vi "Filter_Lowpass - 2D.vi"(1 "Filter":bool caption="Scan", 2 "Input 2D":dbl[][](array[numeric]), 3 "low cutoff freq: fl":dbl=40.0 format="%0.2f") -> (7 "Output":dbl[][](array[numeric]))   [LabVIEW 2018]
uses:
  <vilib>/Analysis/3filter.llb/Filter Passband Type.ctl
  <vilib>/Analysis/4window.llb/windowTd.ctl
  <vilib>/Analysis/3filter.llb/FIR Windowed Filter (DBL).vi
  <vilib>/Analysis/NI_AALBase.lvlib
  <vilib>/Analysis/NI_AALPro.lvlib
  <vilib>/Platform/NI_3dgraph.lvlib
panel:
  in  "3D Surface 2":refnum<k7>(container)
  in  "3D Surface":refnum<k7>(container)
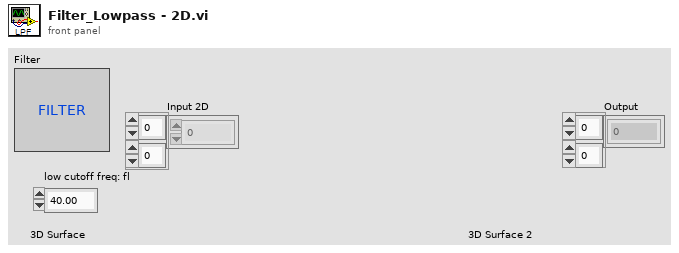
[diagram p1: front panel]
types:
  T1 = typedef "NI_AALBase.lvlib/Filter Passband Type.ctl" = enum32{"Lowpass", "Highpass", "Bandpass", "Bandstop"}
  T2 = typedef "NI_AALPro.lvlib/windowTd.ctl" = u32
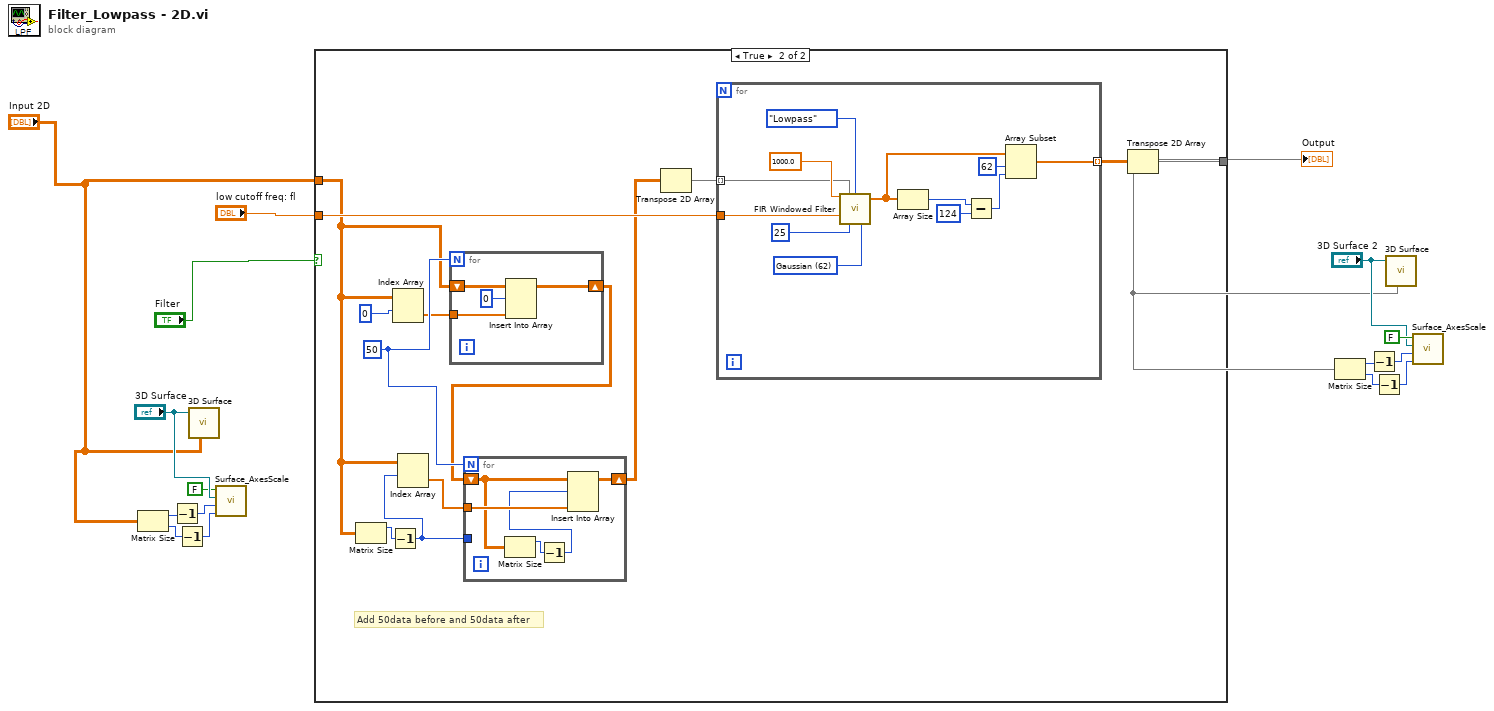
[diagram p0: block diagram]
diagram:
  n1 = Matrix Size(0:"Input 2D") -> (1:w12:i32, 2:w14:i32)
  n2 = Decrement(x=w12) -> (x-1=w10:i32)
  n3 = Decrement(x=w14) -> (x-1=w15:i32)
  n4 = call <vilib>:"3D Surface.vi"("z matrix"="Input 2D", "3D graph"="3D Surface") -> ()  [unwired: 8 in, 2 out]
  n5 = call "Surface_AxesScale.vi"("Y-axis Max"=w15, "X-axis max"=w10, "3D Surface"="3D Surface", "Auto Scale"=FALSE) -> ()  [unwired: 8 in]
  n6 = case shown="True" "Filter" {
    tunnel: "low cutoff freq: fl" -> [_ w30]
    tunnel: "Input 2D" -> [w17 w22]
    tunnel: [w17 w18] -> w1
    frame False {
    }
    frame True {
      w28 = 50
      # "Add 50data before and 50data after"
      n7 = Matrix Size(0:w22) -> (1:w23:i32)  [unwired: 1 out]
      n8 = Decrement(x=w23) -> (x-1=w24:i32)
      n9 = Index Array(array=w22, index (row)=0 ("disabled index (col)")) -> (element=w26:dbl[])  [unwired: 1 in]
      n10 = Index Array(array=w22, index (row)=w24) -> (element=w27:dbl[])  [unwired: 1 in]
      n11 = for {
        N: w28 -> [_]
        shift-right: [w38] -> w21
        shift-left: w22 -> [w39]
        tunnel: w26 -> [w37]
        n12 = Insert Into Array(array=w39, index (row)=0, new element=w37) -> (w38:dbl[][])  [unwired: 1 in]
      }
      n13 = for {
        N: w28 -> [_]
        shift-right: [w35] -> w20
        shift-left: w21 -> [w33]
        tunnel: w27 -> [w34]
        tunnel: w24 -> [_]
        n14 = Matrix Size(0:w33) -> (1:w32:i32)  [unwired: 1 out]
        n15 = Decrement(x=w32) -> (x-1=w31:i32)
        n16 = Insert Into Array(array=w33, index (row)=w31, new element=w34) -> (w35:dbl[][])  [unwired: 1 in]
      }
      n17 = Transpose 2D Array(2D array=w20) -> (transposed array=w19:dbl[][])
      n18 = for {
        tunnel: w30 -> [w44]
        tunnel: w19 -> [w41] mode=indexing
        tunnel: [w42] -> w29 mode=indexing
        w45 = T2 62 items=["Rectangle"=0, "Hanning"=1, "Hamming"=2, "Blackman-Harris"=3, "Exact Blackman"=4, "Blackman"=5, "Flat Top"=6, "4 Term B-Harris "=7, "7 Term B-Harris"=8, "Low Sidelobe"=9, "Blackman Nuttall"=11, "Triangle"=30, "Bartlett-Hanning"=31, "Bohman"=32, "Parzen"=33, "Welch"=34, "Kaiser"=60, "Dolph-Chebyshev"=61, "Gaussian"=62] ("window")
        n19 = call-poly <vilib>:"FIR Windowed Filter.vi"("sampling freq: fs"=1000.0, "X"=w41, "filter type"=Filter_Passband_Type."Lowpass", "low cutoff freq: fl"=w44, "taps"=25, "window"=w45) -> ("Filtered X"=w40:dbl[])  [unwired: 8 in, 1 out]
        n20 = Array Size(array=w40) -> (size(s)=w43:i32)
        n21 = Subtract(x=w43, y=124) -> (x-y=w47:i32)
        n22 = Array Subset(array=w40, index=62, length=w47) -> (w42:dbl[])
      }
      n23 = Transpose 2D Array(2D array=w29) -> (transposed array=w18:dbl[][])
    }
  }
  "Output" <- w1
  n24 = Matrix Size(0:w1) -> (1:w7:i32, 2:w5:i32)
  n25 = Decrement(x=w7) -> (x-1=w9:i32)
  n26 = Decrement(x=w5) -> (x-1=w4:i32)
  n27 = call <vilib>:"3D Surface.vi"("z matrix"=w1, "3D graph"="3D Surface 2") -> ()  [unwired: 8 in, 2 out]
  n28 = call "Surface_AxesScale.vi"("Y-axis Max"=w4, "X-axis max"=w9, "3D Surface"="3D Surface 2", "Auto Scale"=FALSE) -> ()  [unwired: 8 in]
